vi "Periodic Tasks.vi"(8 "error in":errorcluster) -> ()   [LabVIEW 2019]
doc: "This VI runs in parallel to other tasks. It can contain as many user-defined periodic loops as you need. These can carry out PID or other sorts of timed response."
uses:
  <vilib>/Rock Robotics/WPI/ThirdParty/JAS_Junk/TrajLib/Trajectory_Library.lvlib
  Robot Global Data.vi
  <vilib>/Rock Robotics/Network Tables/NT Write Number.vi
  <vilib>/NI_Real-Time Target Support.lvlib
  <vilib>/Rock Robotics/Network Tables/NT Write Boolean.vi
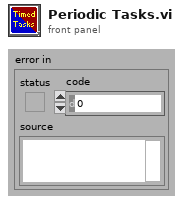
[diagram p1: front panel]
types:
  T1 = typedef "NI_Matrix.lvlib/RealMatrix.ctl" = dbl[][]
  T2 = typedef "Trajectory_Library.lvlib/POSE2D.ctl" = cluster{"TRANSLATION":T3, "ROTATION":T4}
  T3 = typedef "Trajectory_Library.lvlib/TRANSLATION2D.ctl" = cluster{"X":dbl, "Y":dbl}
  T4 = typedef "Trajectory_Library.lvlib/ROTATION2D.ctl" = cluster{"VALUE":dbl, "COS":dbl, "SIN":dbl}
  T5 = typedef "Trajectory_Library.lvlib/DIFF_DRIVE_POSE_EST.ctl" = cluster{"M_VisionContR":T1, "m_nominal_dT":dbl, "m_PrevTime_Sec":dbl, "m_GyroOffset":T4, "m_PrevAngle":T4, "StartLeftEnc_M":dbl, "StartRightEnc_M":dbl, "m_Observer":T6, "m_latencyCompensator":T9}
  T6 = typedef "Trajectory_Library.lvlib/UNSCENTED_KALMAN_FILTER.ctl" = cluster{"m_P":T1, "m_xHat":T1, "States":i32, "Outputs":i32, "m_ContR":T1, "m_ContQ":T1, "m_SigmasF":T1, "m_dT_Sec":dbl, "MERWE_SCALED_SIGMA_PTS":T7, "meanFuncX":T8, "meanFuncY":T8, "residualFuncX":T8, "residualFuncY":T8, "addFuncX":T8, "addFuncXExtra":variant, "residualFuncYExtra":variant, "residualFuncXExtra":variant, "MeanFuncYExtra":variant, "MeanFuncXExtra":variant, "Inputs":i32}
  T7 = typedef "Trajectory_Library.lvlib/MERWE_SCALED_SIGMA_PTS.ctl" = cluster{"m_Wm":T1, "States":i32, "Alpha":dbl, "m_Wc":T1, "Kappa":i32}
  T8 = typedef "Trajectory_Library.lvlib/CALLBACK_FUNC_TYPE.ctl" = refnum<vi>
  T9 = typedef "Trajectory_Library.lvlib/KALMAN_FILTER_LATENCY_COMP.ctl" = cluster{"m_pastObserverSnapshots ":T10[]}
  T10 = typedef "Trajectory_Library.lvlib/OBSERVER_SNAP_LIST_ITEM.ctl" = cluster{"TimeStamp":dbl, "OBSERVER_SNAPSHOT":T11}
  T11 = typedef "Trajectory_Library.lvlib/OBSERVER_SNAPSHOT.ctl" = cluster{"ErrorCoVariance":T1, "xHat":T1, "LocalMeasurements":T1, "Inputs":T1}
  T12 = enum16{"Moving Average", "Low Pass 1st Order Butterworth", "Low Pass 2nd Order Butterworth", "High Pass 1st Order Butterworth", "High Pass 2nd Order Butterworth"}
  T13 = typedef "NI_Real-Time Target Support.lvlib/RT CPU Load.ctl" = cluster{"Total (%)":dbl, "Time Critical (%)":dbl, "Timed Structures (%)":dbl, "High (%)":dbl, "Above Normal (%)":dbl, "Normal (%)":dbl, "Background (%)":dbl, "Idle (%)":dbl, "ISR (%)":dbl}
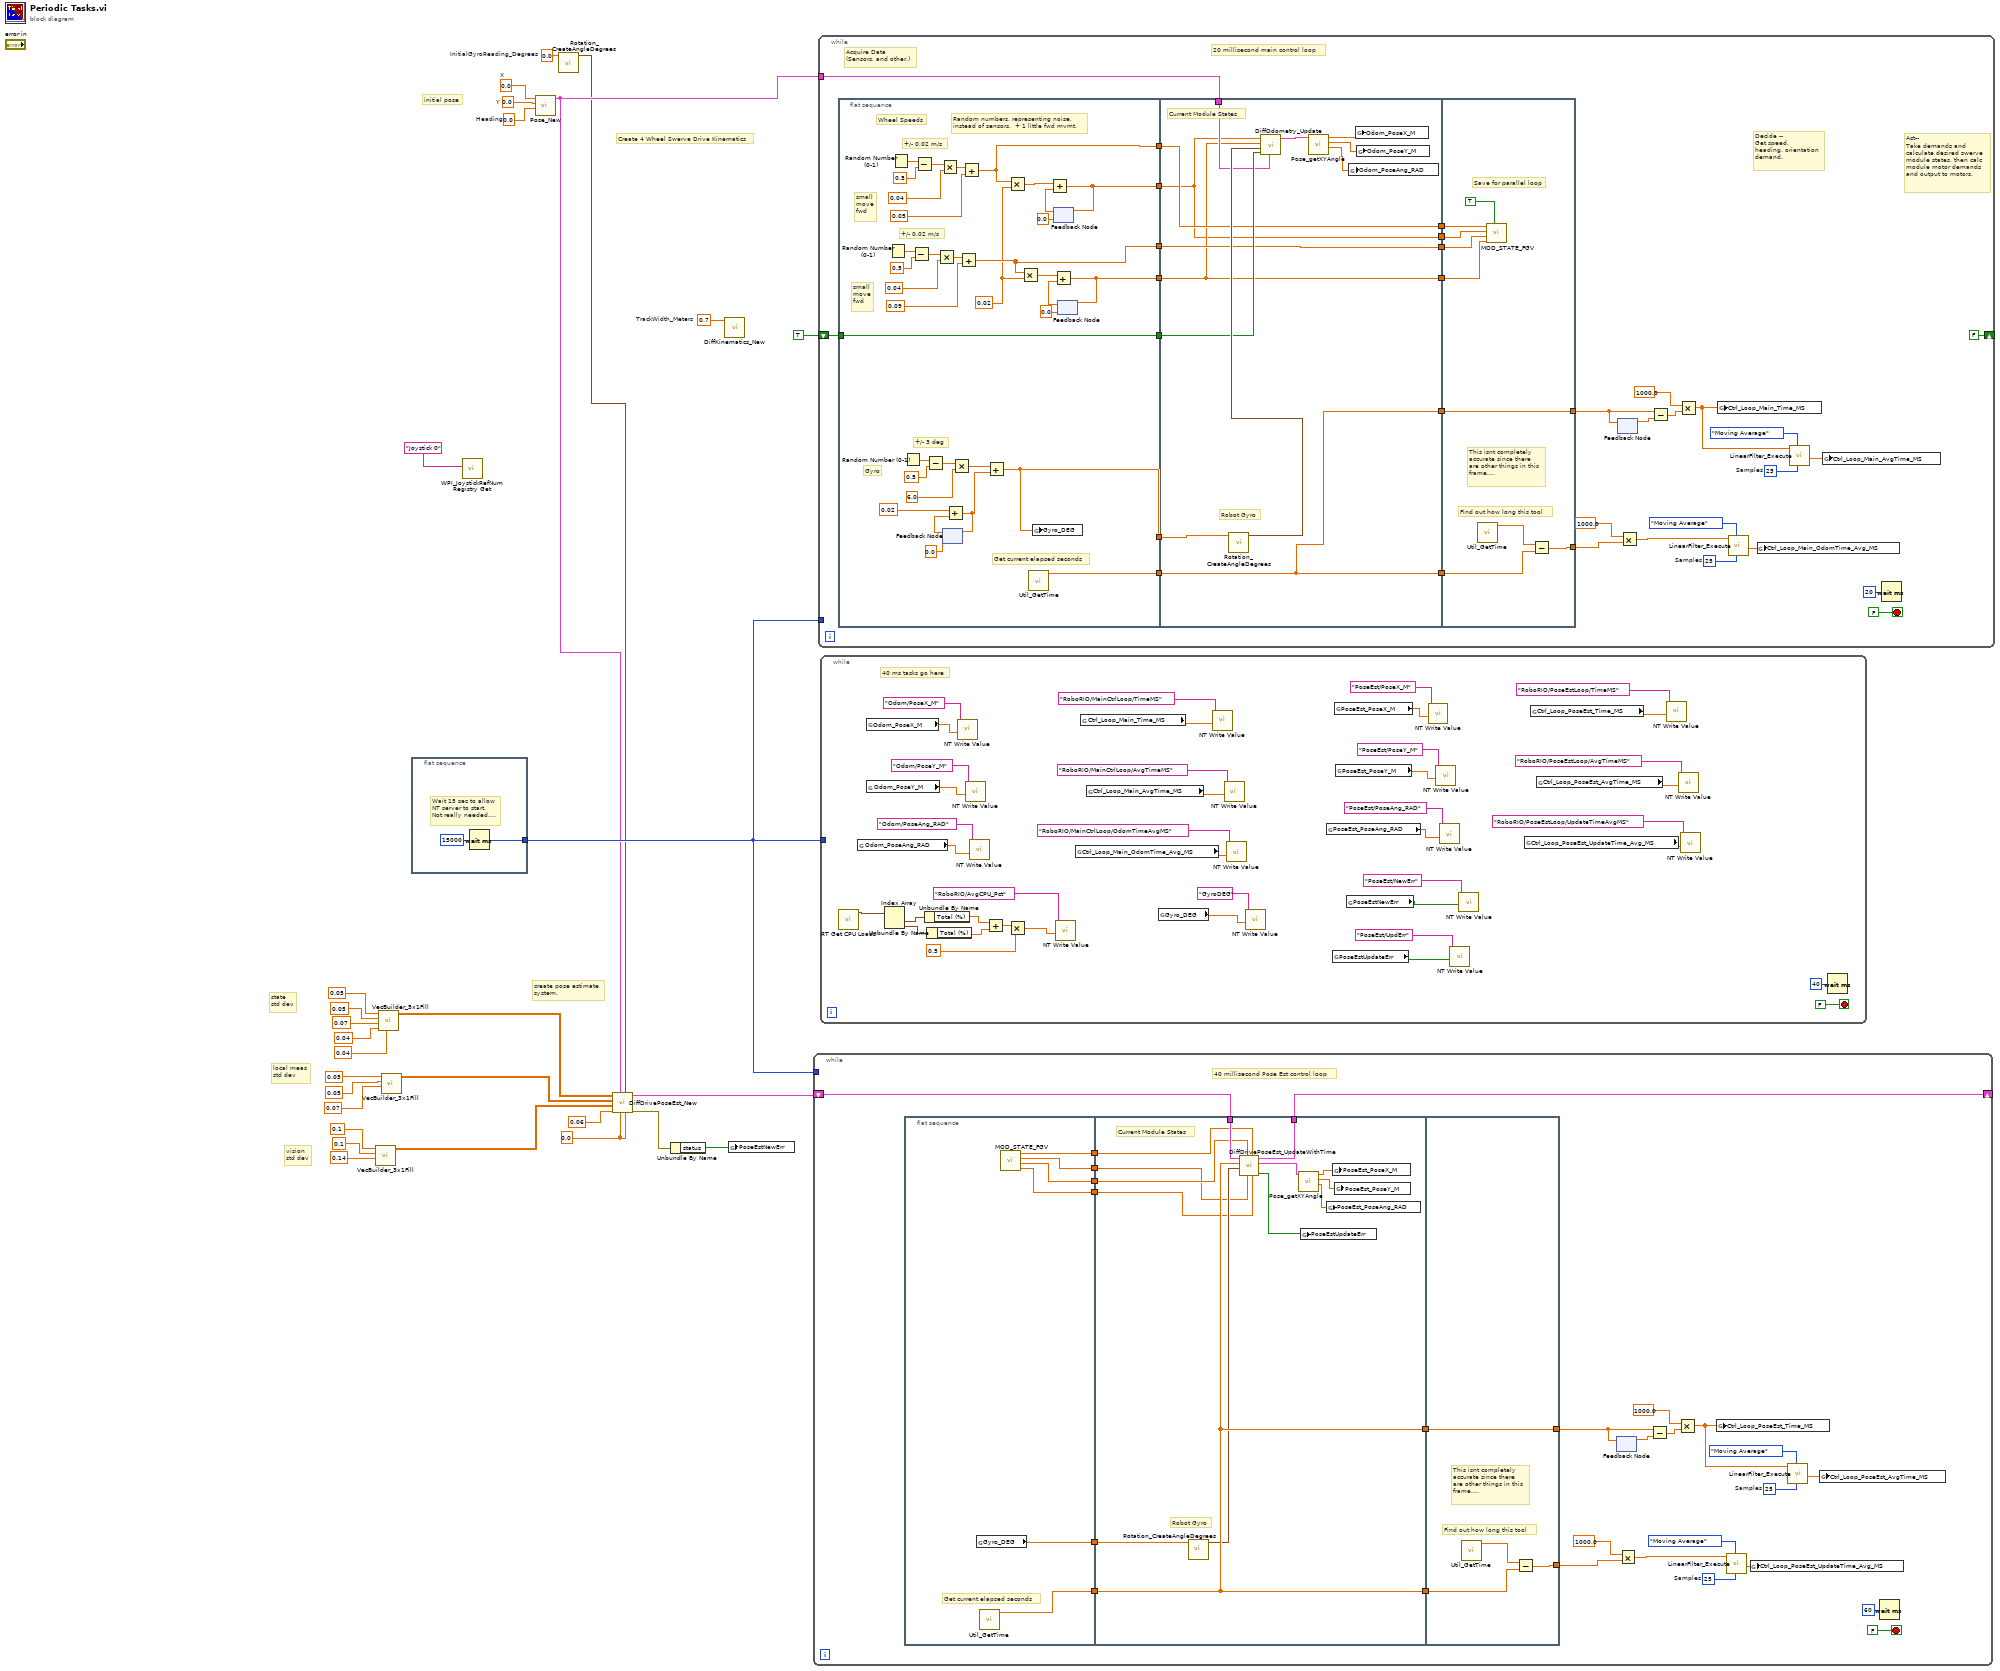
[diagram p0: block diagram]
diagram:
  w9 = 0.0 ("LeftDistance_M")
  w16 = 0.7  # TrackWidth_Meters
  w25 = 0.0  # X
  w26 = 0.0  # Y
  w27 = 0.0  # Heading
  w28 = 0.0  # InitialGyroReading_Degrees
  # "vision \nstd dev"
  # "local meas\nstd dev"
  # "state\nstd dev"
  # "create pose estimate\nsystem."
  # "initial pose"
  # "Create 4 Wheel Swerve Drive Kinematics"
  n1 = call <vilib>:"VecBuilder_3x1Fill.vi"("R2"=0.14 ("element"), "R1"=0.1 ("element"), "R0"=0.1 ("element")) -> ("output matrix"=w11:T1)  [unwired: 8 in]
  n2 = call <vilib>:"VecBuilder_5x1Fill.vi"("R4"=0.04, "R3"=0.04, "R2"=0.07 ("element"), "R1"=0.05 ("element"), "R0"=0.05 ("element")) -> ("output matrix"=w13:T1)  [unwired: 6 in]
  n3 = call <vilib>:"VecBuilder_3x1Fill.vi"("R2"=0.07 ("element"), "R1"=0.05 ("element"), "R0"=0.05 ("element")) -> ("output matrix"=w12:T1)  [unwired: 8 in]
  n4 = flat-sequence {
    tunnel: [w30] -> w17
    frame #0 {
      # "Wait 15 sec to allow\nNT server to start.\nNot really needed...."
      n5 = Wait (ms)(milliseconds to wait=u32 15000) -> (millisecond timer value=w30:u32)
    }
  }
  n6 = call <vilib>:"WPI_JoystickRefNum Registry Get.vi"("refnum name"="Joystick 0") -> ()  [unwired: 1 in, 10 out]
  n7 = call <vilib>:"Pose_New.vi"("Heading"=w27, "Y"=w26, "X"=w25) -> ("out POSe"=w14:T2)  [unwired: 8 in]
  n8 = call <vilib>:"Rotation_CreateAngleDegrees.vi"("Angle_Degrees"=w28) -> ("ROTATION"=w7:T4)  [unwired: 10 in]
  n9 = call <vilib>:"DiffDrivePoseEst_New.vi"("RightDistance_M"=w9, "gyroAngle"=w7, "LeftDistance_M"=w9, "InitialPose"=w14, "dt_Seconds"=0.06, "VisionMeasurementStdDevs"=w11, "LocalMeasurementStdDevs"=w12, "StateStdDevs"=w13) -> ("Error"=w2:errorcluster, "DiffDrivePoseEstimate"=w8:T5)  [unwired: 2 in]
  n10 = Unbundle By Name(w2) -> ("status"=w1:bool)
  n11 = call <vilib>:"DiffKinematics_New.vi"("TrackWidth_Meters"=w16) -> ()  [unwired: 10 in, 1 out]
  n12 = global write "Robot Global Data.vi" "PoseEstNewErr"(w1) -> ()
  n13 = while {
    shift-right: [w32] -> _
    shift-left: w8 -> [w55]
    tunnel: w17 -> [_]
    stop <- FALSE stop-if-true
    w41 = 25  # Samples
    w51 = 25  # Samples
    # "40 millisecond Pose Est control loop"
    n14 = flat-sequence {
      tunnel: [w63] -> w46
      tunnel: [w62] -> w37
      tunnel: [w61] -> w36
      tunnel: [w60] -> w35
      tunnel: [w59] -> w34
      tunnel: [w58] -> w33
      tunnel: w55 -> [w71]
      tunnel: w46 -> [w68]
      tunnel: [w68] -> w45
      tunnel: [w68] -> w44
      tunnel: w37 -> [w70]
      tunnel: w36 -> [w66]
      tunnel: w35 -> [w69]
      tunnel: w34 -> [w65]
      tunnel: w33 -> [w74]
      tunnel: [w72] -> w32
      tunnel: [w81] -> w47
      tunnel: w45 -> [w81]
      tunnel: w44 -> [w79]
      tunnel: [w78] -> w42
      frame #0 {
        # "Get current elapsed seconds"
        n15 = global read "Robot Global Data.vi" "Gyro_DEG"() -> (w58:dbl)
        n16 = call <vilib>:"Util_GetTime.vi"() -> ("FPGA_Time_Seconds"=w63:dbl)  [unwired: 10 in, 1 out]
        n17 = call "MOD_STATE_FGV.vi"() -> ("out Right Dist"=w59:dbl, "out Right Speed"=w60:dbl, "out Left Dist"=w61:dbl, "out Left Speed"=w62:dbl)  [unwired: 8 in]
      }
      frame #1 {
        # "Current Module States"
        # "Robot Gyro"
        n18 = call <vilib>:"Rotation_CreateAngleDegrees.vi"("Angle_Degrees"=w74) -> ("ROTATION"=w67:T4)  [unwired: 10 in]
        n19 = call <vilib>:"DiffDrivePoseEst_UpdateWithTime.vi"("RightDistance"=w65, "LeftSpeed"=w70, "LeftDistance"=w66, "RightSpeed"=w69, "GyroAngle"=w67, "CurrentTimeSeconds"=w68, "in DiffDrivePoseEstimate"=w71) -> ("Error"=w64:bool, "Estimated Pose"=w73:T2, "Out DiffDrivePoseEstimate"=w72:T5)  [unwired: 2 in]
        n20 = call <vilib>:"Pose_getXYAngle.vi"("in POSE"=w73) -> ("Angle"=w75:dbl, "Y"=w76:dbl, "X"=w77:dbl)  [unwired: 8 in]
        n21 = global write "Robot Global Data.vi" "PoseEstUpdateErr"(w64) -> ()
        n22 = global write "Robot Global Data.vi" "PoseEst_PoseAng_RAD"(w75) -> ()
        n23 = global write "Robot Global Data.vi" "PoseEst_PoseX_M"(w77) -> ()
        n24 = global write "Robot Global Data.vi" "PoseEst_PoseY_M"(w76) -> ()
      }
      frame #2 {
        # "This isnt completely\naccurate since there\nare other things in this\nframe...."
        # "Find out how long this tool"
        n25 = call <vilib>:"Util_GetTime.vi"() -> ("FPGA_Time_Seconds"=w80:dbl)  [unwired: 10 in, 1 out]
        n26 = Subtract(x=w80, y=w79) -> (x-y=w78:dbl)
      }
    }
    n27 = feedback-in #1(w47) -> ()
    n28 = feedback #1() -> (w54:dbl)  [unwired: 1 in]
    n29 = Multiply(x=1000.0, y=w42) -> (x*y=w39:dbl)
    n30 = Subtract(x=w47, y=w54) -> (x-y=w53:dbl)
    n31 = Multiply(x=1000.0, y=w53) -> (x*y=w49:dbl)
    n32 = global write "Robot Global Data.vi" "Ctrl_Loop_PoseEst_Time_MS"(w49) -> ()
    n33 = call <vilib>:"LinearFilter_Execute.vi"("Samples"=w41, "Filter Type"=T12."Moving Average", "Input"=w39) -> ("Output"=w38:dbl)  [unwired: 7 in, 1 out]
    n34 = global write "Robot Global Data.vi" "Ctrl_Loop_PoseEst_UpdateTime_Avg_MS"(w38) -> ()
    n35 = call <vilib>:"LinearFilter_Execute.vi"("Samples"=w51, "Filter Type"=T12."Moving Average", "Input"=w49) -> ("Output"=w48:dbl)  [unwired: 7 in, 1 out]
    n36 = global write "Robot Global Data.vi" "Ctrl_Loop_PoseEst_AvgTime_MS"(w48) -> ()
    n37 = Wait (ms)(milliseconds to wait=u32 60) -> ()  [unwired: 1 out]
  }
  n38 = while {
    tunnel: w17 -> [_]
    shift-right: [FALSE] -> _
    shift-left: TRUE -> [w88]
    tunnel: w14 -> [w87]
    stop <- FALSE stop-if-true
    w95 = 25  # Samples
    w108 = 25  # Samples
    # "Act--\nTake demands and \ncalculate desired swerve\nmodule states, then calc\nmodule motor demands\nand output to motors."
    # "Decide -- \nGet speed,\nheading, orientation\ndemand."
    # "Acquire Data\n(Sensors, and other.)"
    # "20 millisecond main control loop"
    n39 = flat-sequence {
      tunnel: [w118] -> w103
      tunnel: [w148] -> w102
      tunnel: [w131] -> w101
      tunnel: [w130] -> w100
      tunnel: [w122] -> w91
      tunnel: [w121] -> w90
      tunnel: [w120] -> w89
      tunnel: w88 -> [w120]
      tunnel: w103 -> [w161]
      tunnel: w102 -> [w160]
      tunnel: w101 -> [w152]
      tunnel: w100 -> [w151]
      tunnel: [w160] -> w99
      tunnel: [w160] -> w98
      tunnel: w91 -> [w149]
      tunnel: w90 -> [w150]
      tunnel: w89 -> [w154]
      tunnel: w87 -> [w153]
      tunnel: [w152] -> w86
      tunnel: [w149] -> w85
      tunnel: [w151] -> w84
      tunnel: [w150] -> w83
      tunnel: [w170] -> w104
      tunnel: w99 -> [w170]
      tunnel: w98 -> [w167]
      tunnel: [w166] -> w96
      tunnel: w86 -> [w165]
      tunnel: w85 -> [w164]
      tunnel: w84 -> [w163]
      tunnel: w83 -> [w162]
      frame #0 {
        w129 = 0.02 ("y")
        # "small\nmove\nfwd"
        # "+/- 0.02 m/s"
        # "small\nmove\nfwd"
        # "+/- 0.02 m/s"
        # "Wheel Speeds"
        # "Random numbers, representing noise,\ninstead of sensors.  + 1 little fwd mvmt."
        # "Gyro"
        # "+/- 3 deg"
        # "Get current elapsed seconds"
        n40 = Random Number (0-1)() -> (number: 0 to 1=w141:dbl)
        n41 = Random Number (0-1)() -> (number: 0 to 1=w138:dbl)
        n42 = Random Number (0-1)() -> (number: 0 to 1=w146:dbl)
        n43 = Subtract(x=w141, y=0.5) -> (x-y=w142:dbl)
        n44 = Subtract(x=w138, y=0.5) -> (x-y=w139:dbl)
        n45 = Subtract(x=w146, y=0.5) -> (x-y=w147:dbl)
        n46 = Multiply(x=w142, y=0.04) -> (x*y=w143:dbl)
        n47 = Multiply(x=w139, y=0.04) -> (x*y=w140:dbl)
        n48 = feedback #2(0.0) -> (w115:dbl)
        n49 = Add(x=0.02 ("y"), y=w115) -> (x+y=w116:dbl)
        n50 = feedback-in #2(w116) -> ()
        n51 = Multiply(x=w147, y=6.0) -> (x*y=w119:dbl)
        n52 = Add(x=w143, y=0.09) -> (x+y=w130:dbl)
        n53 = Add(x=w140, y=0.05) -> (x+y=w131:dbl)
        n54 = Add(x=w119, y=w116) -> (x+y=w118:dbl)
        n55 = Multiply(x=w131, y=w129) -> (x*y=w123:dbl)
        n56 = Multiply(x=w130, y=w129) -> (x*y=w128:dbl)
        n57 = call <vilib>:"Util_GetTime.vi"() -> ("FPGA_Time_Seconds"=w148:dbl)  [unwired: 10 in, 1 out]
        n58 = global write "Robot Global Data.vi" "Gyro_DEG"(w118) -> ()
        n59 = feedback #3(0.0) -> (w125:dbl)
        n60 = Add(x=w123, y=w125) -> (x+y=w122:dbl)
        n61 = feedback-in #3(w122) -> ()
        n62 = feedback #4(0.0) -> (w127:dbl)
        n63 = Add(x=w128, y=w127) -> (x+y=w121:dbl)
        n64 = feedback-in #4(w121) -> ()
      }
      frame #1 {
        # "Current Module States"
        # "Robot Gyro"
        n65 = call <vilib>:"Rotation_CreateAngleDegrees.vi"("Angle_Degrees"=w161) -> ("ROTATION"=w155:T4)  [unwired: 10 in]
        n66 = call <vilib>:"DiffOdometry_Update.vi"("Reset Pose"=w153, "Reset"=w154, "Heading"=w155, "RightDistance"=w150, "LeftDistance"=w149) -> ("CurrentRelativePose"=w159:T2)  [unwired: 6 in]
        n67 = call <vilib>:"Pose_getXYAngle.vi"("in POSE"=w159) -> ("Angle"=w156:dbl, "Y"=w157:dbl, "X"=w158:dbl)  [unwired: 8 in]
        n68 = global write "Robot Global Data.vi" "Odom_PoseAng_RAD"(w156) -> ()
        n69 = global write "Robot Global Data.vi" "Odom_PoseX_M"(w158) -> ()
        n70 = global write "Robot Global Data.vi" "Odom_PoseY_M"(w157) -> ()
      }
      frame #2 {
        # "This isnt completely\naccurate since there\nare other things in this\nframe...."
        # "Find out how long this tool"
        # "Save for parallel loop"
        n71 = call <vilib>:"Util_GetTime.vi"() -> ("FPGA_Time_Seconds"=w168:dbl)  [unwired: 10 in, 1 out]
        n72 = call "MOD_STATE_FGV.vi"("Write"=TRUE, "Right Dist"=w162, "Right Speed"=w163, "Left Dist"=w164, "Left Speed"=w165) -> ()  [unwired: 3 in, 4 out]
        n73 = Subtract(x=w168, y=w167) -> (x-y=w166:dbl)
      }
    }
    n74 = feedback-in #5(w104) -> ()
    n75 = feedback #5() -> (w111:dbl)  [unwired: 1 in]
    n76 = Multiply(x=1000.0, y=w96) -> (x*y=w93:dbl)
    n77 = Subtract(x=w104, y=w111) -> (x-y=w110:dbl)
    n78 = Multiply(x=1000.0, y=w110) -> (x*y=w106:dbl)
    n79 = global write "Robot Global Data.vi" "Ctrl_Loop_Main_Time_MS"(w106) -> ()
    n80 = call <vilib>:"LinearFilter_Execute.vi"("Samples"=w95, "Filter Type"=T12."Moving Average", "Input"=w93) -> ("Output"=w92:dbl)  [unwired: 7 in, 1 out]
    n81 = global write "Robot Global Data.vi" "Ctrl_Loop_Main_OdomTime_Avg_MS"(w92) -> ()
    n82 = call <vilib>:"LinearFilter_Execute.vi"("Samples"=w108, "Filter Type"=T12."Moving Average", "Input"=w106) -> ("Output"=w105:dbl)  [unwired: 7 in, 1 out]
    n83 = global write "Robot Global Data.vi" "Ctrl_Loop_Main_AvgTime_MS"(w105) -> ()
    n84 = Wait (ms)(milliseconds to wait=u32 20) -> ()  [unwired: 1 out]
  }
  n85 = while {
    tunnel: w17 -> [_]
    stop <- FALSE stop-if-true
    # "40 ms tasks go here"
    n86 = call <vilib>:"RT Get CPU Loads.vi"() -> ("CPU loads"=w203:T13[])  [unwired: 10 in, 1 out]
    n87 = global read "Robot Global Data.vi" "Odom_PoseAng_RAD"() -> (w204:dbl)
    n88 = global read "Robot Global Data.vi" "Odom_PoseX_M"() -> (w208:dbl)
    n89 = global read "Robot Global Data.vi" "Odom_PoseY_M"() -> (w205:dbl)
    n90 = Index Array(array=w203) -> (element #1=w202:T13, element #2=w201:T13)  [unwired: 2 in]
    n91 = Unbundle By Name(w202) -> ("Total (%)"=w200:dbl)
    n92 = Unbundle By Name(w201) -> ("Total (%)"=w199:dbl)
    n93 = call-poly <vilib>:"NT Write Value.vi"("Numeric"=w208, "Name"="Odom/PoseX_M") -> ()  [unwired: 9 in, 1 out]
    n94 = call-poly <vilib>:"NT Write Value.vi"("Numeric"=w205, "Name"="Odom/PoseY_M") -> ()  [unwired: 9 in, 1 out]
    n95 = call-poly <vilib>:"NT Write Value.vi"("Numeric"=w204, "Name"="Odom/PoseAng_RAD") -> ()  [unwired: 9 in, 1 out]
    n96 = Add(x=w200, y=w199) -> (x+y=w198:dbl)
    n97 = Multiply(x=w198, y=0.5) -> (x*y=w195:dbl)
    n98 = call-poly <vilib>:"NT Write Value.vi"("Numeric"=w195, "Name"="RoboRIO/AvgCPU_Pct") -> ()  [unwired: 9 in, 1 out]
    n99 = global read "Robot Global Data.vi" "Ctrl_Loop_Main_OdomTime_Avg_MS"() -> (w189:dbl)
    n100 = global read "Robot Global Data.vi" "Ctrl_Loop_Main_Time_MS"() -> (w193:dbl)
    n101 = global read "Robot Global Data.vi" "Ctrl_Loop_Main_AvgTime_MS"() -> (w191:dbl)
    n102 = global read "Robot Global Data.vi" "Gyro_DEG"() -> (w171:dbl)
    n103 = call-poly <vilib>:"NT Write Value.vi"("Numeric"=w193, "Name"="RoboRIO/MainCtrlLoop/TimeMS") -> ()  [unwired: 9 in, 1 out]
    n104 = call-poly <vilib>:"NT Write Value.vi"("Numeric"=w191, "Name"="RoboRIO/MainCtrlLoop/AvgTimeMS") -> ()  [unwired: 9 in, 1 out]
    n105 = call-poly <vilib>:"NT Write Value.vi"("Numeric"=w189, "Name"="RoboRIO/MainCtrlLoop/OdomTimeAvgMS") -> ()  [unwired: 9 in, 1 out]
    n106 = call-poly <vilib>:"NT Write Value.vi"("Numeric"=w171, "Name"="GyroDEG") -> ()  [unwired: 9 in, 1 out]
    n107 = global read "Robot Global Data.vi" "PoseEst_PoseAng_RAD"() -> (w183:dbl)
    n108 = global read "Robot Global Data.vi" "PoseEstUpdateErr"() -> (w173:bool)
    n109 = global read "Robot Global Data.vi" "PoseEst_PoseX_M"() -> (w187:dbl)
    n110 = global read "Robot Global Data.vi" "PoseEst_PoseY_M"() -> (w184:dbl)
    n111 = global read "Robot Global Data.vi" "PoseEstNewErr"() -> (w175:bool)
    n112 = call-poly <vilib>:"NT Write Value.vi"("Numeric"=w187, "Name"="PoseEst/PoseX_M") -> ()  [unwired: 9 in, 1 out]
    n113 = call-poly <vilib>:"NT Write Value.vi"("Numeric"=w184, "Name"="PoseEst/PoseY_M") -> ()  [unwired: 9 in, 1 out]
    n114 = call-poly <vilib>:"NT Write Value.vi"("Numeric"=w183, "Name"="PoseEst/PoseAng_RAD") -> ()  [unwired: 9 in, 1 out]
    n115 = call-poly <vilib>:"NT Write Value.vi"("Boolean"=w173, "Name"="PoseEst/UpdErr") -> ()  [unwired: 9 in, 1 out]
    n116 = call-poly <vilib>:"NT Write Value.vi"("Boolean"=w175, "Name"="PoseEst/NewErr") -> ()  [unwired: 9 in, 1 out]
    n117 = global read "Robot Global Data.vi" "Ctrl_Loop_PoseEst_UpdateTime_Avg_MS"() -> (w177:dbl)
    n118 = global read "Robot Global Data.vi" "Ctrl_Loop_PoseEst_Time_MS"() -> (w181:dbl)
    n119 = global read "Robot Global Data.vi" "Ctrl_Loop_PoseEst_AvgTime_MS"() -> (w179:dbl)
    n120 = call-poly <vilib>:"NT Write Value.vi"("Numeric"=w181, "Name"="RoboRIO/PoseEstLoop/TimeMS") -> ()  [unwired: 9 in, 1 out]
    n121 = call-poly <vilib>:"NT Write Value.vi"("Numeric"=w179, "Name"="RoboRIO/PoseEstLoop/AvgTimeMS") -> ()  [unwired: 9 in, 1 out]
    n122 = call-poly <vilib>:"NT Write Value.vi"("Numeric"=w177, "Name"="RoboRIO/PoseEstLoop/UpdateTimeAvgMS") -> ()  [unwired: 9 in, 1 out]
    n123 = Wait (ms)(milliseconds to wait=u32 40) -> ()  [unwired: 1 out]
  }
